vi "round.step.10.11.12.13.vi"(8 "E.Values":u64[][](array[numeric]), 9 "D.Values":u64[](array[numeric]), 10 "D.Offsets":i32, 11 "Left Shifts":i32[](array[numeric])) -> (3 "Final.A.Out":u64[](array[numeric]))   [LabVIEW 2021]
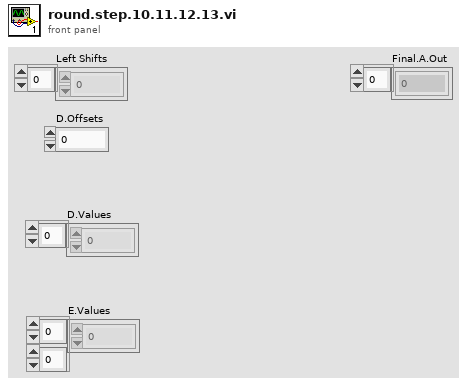
[diagram p1: front panel]
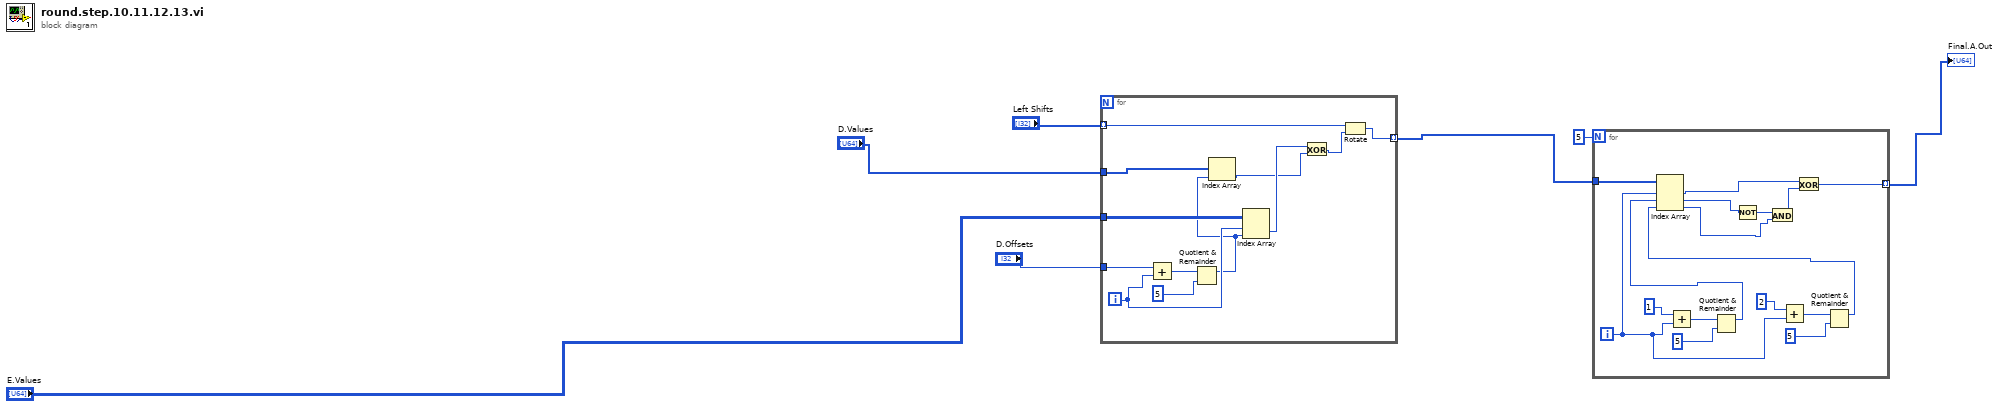
[diagram p0: block diagram]
diagram:
  n1 = for {
    tunnel: "E.Values" -> [w19]
    tunnel: [w15] -> w4 mode=indexing
    tunnel: "Left Shifts" -> [w16] mode=indexing
    tunnel: "D.Values" -> [w11]
    tunnel: "D.Offsets" -> [w8]
    i -> [w13]
    n2 = Add(x=w8, y=w13) -> (x+y=w18:i32)
    n3 = Quotient & Remainder(x=w18, y=5 ("x")) -> (x-y*floor(x/y)=w10:i32)  [unwired: 1 out]
    n4 = Index Array(array=w11, index=w10) -> (element=w9:u64)
    n5 = Index Array(array=w19, index (row)=w13, index (col)=w10) -> (element=w12:u64)
    n6 = Exclusive Or(1:w9, 2:w12) -> (0:w14:u64)
    n7 = Rotate(1:w14, 2:w16) -> (0:w15:u64)
  }
  n8 = for {
    N: 5 -> [_]
    tunnel: w4 -> [w32]
    tunnel: [w20] -> w5 mode=indexing
    i -> [w22]
    n9 = Add(x=1, y=w22) -> (x+y=w34:i32)
    n10 = Quotient & Remainder(x=w34, y=5 ("x")) -> (x-y*floor(x/y)=w26:i32)  [unwired: 1 out]
    n11 = Add(x=2, y=w22) -> (x+y=w24:i32)
    n12 = Quotient & Remainder(x=w24, y=5 ("x")) -> (x-y*floor(x/y)=w21:i32)  [unwired: 1 out]
    n13 = Index Array(array=w32, index #1=w22, index #2=w26, index #3=w21) -> (element #1=w31:u64, element #2=w28:u64, element #3=w27:u64)
    n14 = Not(x=w28) -> (.not. x?=w30:u64)
    n15 = And(x=w30, y=w27) -> (x .and. y?=w29:u64)
    n16 = Exclusive Or(1:w29, 2:w31) -> (0:w20:u64)
  }
  "Final.A.Out" <- w5
